vi "Find.vi"(7 "default":refnum<class "Plugin Thread.lvclass">, 8 "error in (no error)":errorcluster, 11 "Components":refnum<class "Component.lvclass">[](array[class])) -> (0 "error out":errorcluster, 2 "found?":bool, 3 "Plugin Thread":refnum<class "Plugin Thread.lvclass">)   [LabVIEW 2020, in "DSF Core.lvlib" / "Plugin Thread.lvclass"]
uses:
  Plugin Thread.lvclass
  Component/Component.lvclass
  Component/Component.lvclass/Component.ctl
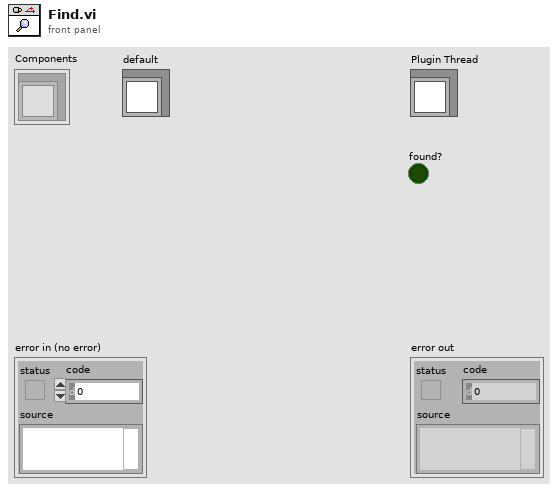
[diagram p1: front panel]
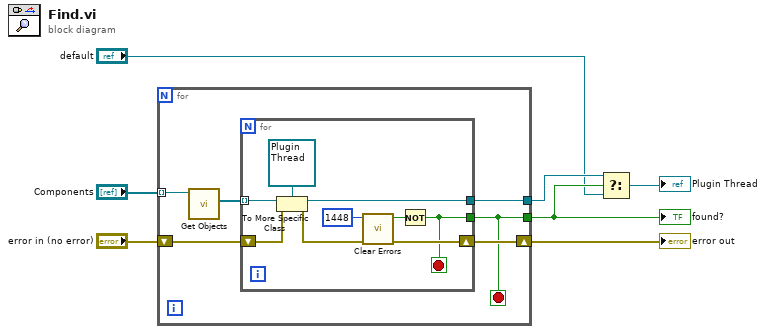
[diagram p0: block diagram]
diagram:
  n1 = for {
    tunnel: "Components" -> [w10] mode=indexing
    tunnel: [w12] -> w3
    tunnel: [w8] -> w4
    shift-right: [w11] -> w5
    shift-left: "error in (no error)" -> [w13]
    stop <- w8 stop-if-true
    n2 = call "Get Objects.vi"("Component in"=w10) -> ("objects"=w9:refnum<class>[])  [unwired: 9 in, 1 out]
    n3 = for {
      tunnel: w9 -> [w21] mode=indexing
      shift-right: [w18] -> w11
      shift-left: w13 -> [w17]
      tunnel: [w15] -> w8
      tunnel: [w14] -> w12
      stop <- w15 stop-if-true
      n4 = To More Specific Class(target class=refnum<class "Plugin Thread.lvclass"> refnum ("DSF.Engine.lvlib:Transceiver"), reference=w21, error in=w17) -> (specific class reference=w14:refnum<class "Plugin Thread.lvclass">, error out=w19:errorcluster)
      n5 = call <vilib>:"Clear Errors.vi"("error in (no error)"=w19, "specific error code to clear (0: all)"=1448) -> ("error out"=w18:errorcluster, "specific error cleared?"=w16:bool)  [unwired: 4 in]
      n6 = Not(x=w16) -> (.not. x?=w15:bool)
    }
  }
  "error out" <- w5
  "found?" <- w4
  n7 = Select(t=w3, s=w4, f="default") -> (s? t:f=→"Plugin Thread":refnum<class "Plugin Thread.lvclass">)
